vi "Battery Level Test.vi"   [LabVIEW 2013]
uses:
  <vilib>/Rock Robotics/SystemInterfaces/Typedef/FPGA_TypedefAnalogModule.ctl
  <vilib>/Rock Robotics/SystemInterfaces/AI/FPGA_AIChannel.ctl
  <vilib>/Rock Robotics/SystemInterfaces/Typedef/FPGA_TypedefDigitalModule.ctl
types:
  T1 = typedef "FPGA_AIChannel.ctl" = enum8{"AI 1", "AI 2", "AI 3", "AI 4", "AI 5", "AI 6", "AI 7", "AI 8", "Invalid"}
  T2 = typedef "FPGA_TypedefAnalogModule.ctl" = enum16{"Analog Module 1", "Analog Module 2"}
  T3 = typedef "WPI_AnalogChannelDevRef.ctl" = cluster{"DevStatus":errorcluster, "Analog Module":T2, "Analog Channel":T1}
  T4 = typedef "FPGA_TypedefDigitalModule.ctl" = enum16{"Digital Module 1", "Digital Module 2"}
  T5 = enum16{"FOUR_ZONES", "ONE_ZONE_TWO_LINES", "TWO_ZONES_ONE_LINE"}
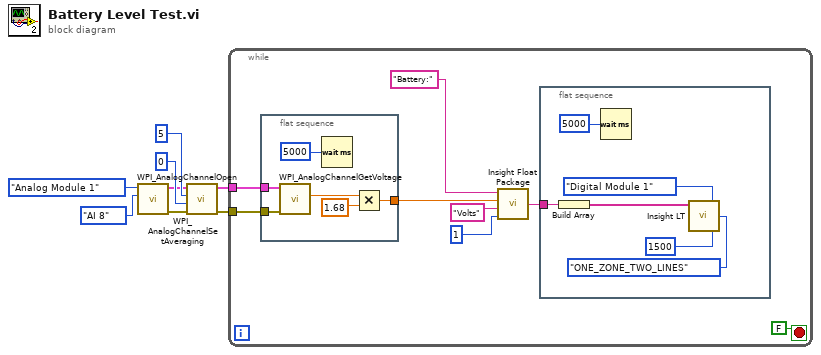
[diagram p0: block diagram]
diagram:
  n1 = call <vilib>:"WPI_AnalogChannelOpen.vi"("Analog Channel"=FPGA_AIChannel."AI 8", "Analog Module (Module 1)"=FPGA_TypedefAnalogModule."Analog Module 1") -> ("error out"=w4:errorcluster, "AIDeviceRef"=w3:T3)  [unwired: 8 in]
  n2 = call <vilib>:"WPI_AnalogChannelSetAveraging.vi"("error in (no error)"=w4, "OversampleBits"=u8 0, "AverageBits"=u8 5, "AIDeviceRef"=w3) -> ("error out"=w1:errorcluster, "AIDeviceRef"=w2:T3)  [unwired: 6 in]
  n3 = while {
    tunnel: w1 -> [w15]
    tunnel: w2 -> [w14]
    stop <- FALSE stop-if-true
    n4 = flat-sequence {
      tunnel: w15 -> [w26]
      tunnel: w14 -> [w25]
      tunnel: [w24] -> w12
      frame #0 {
        n5 = call <vilib>:"WPI_AnalogChannelGetVoltage.vi"("error in (no error)"=w26, "AIDeviceRef"=w25) -> ("Voltage"=w28:dbl)  [unwired: 7 in, 2 out]
        n6 = Wait (ms)(milliseconds to wait=u32 5000) -> ()  [unwired: 1 out]
        n7 = Multiply(x=w28, y=1.68) -> (x*y=w24:dbl)
      }
    }
    n8 = call "Insight Float Package.vi"("Decimal Places"=1, "Footer"="Volts", "Float"=w12, "Header"="Battery:") -> ("resulting string"=w13:string)
    n9 = flat-sequence {
      tunnel: w13 -> [w22]
      frame #0 {
        n10 = Build Array(w22) -> (w21:string[])
        n11 = Wait (ms)(milliseconds to wait=u32 5000) -> ()  [unwired: 1 out]
        n12 = call "Insight LT.vi"("Scroll Timing"=1500, "ZONE \nCONFIGURATION"=T5."ONE_ZONE_TWO_LINES" ("ZONE \nCONFIGURATION"), "Digital Module"=FPGA_TypedefDigitalModule."Digital Module 1", "Zone 1 Data"=w21) -> ()  [unwired: 3 in]
      }
    }
  }
